vi "tokenizer.vi"() -> ()   [LabVIEW 2016]
uses:
  <vilib>/regexp/Match Regular Expression.xnode
panel:
  in  "input YAML":string
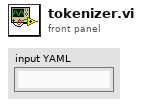
[diagram p1: front panel]
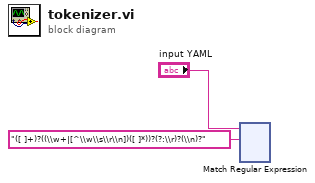
[diagram p0: block diagram]
diagram:
  n1 = xnode "Match Regular Expression"("input string"="input YAML", "regular expression"="([ ]+)?((\\w+|[^\\w\\s\\r\\n])([ ]*))?(?:\\r)?(\\n)?") -> ()  [unwired: 4 in, 5 out]
